vi "NormalToHex.vi"(11 "Input":string="1234") -> (3 "Output":string)   [LabVIEW 2013, in "main.lvlib"]
uses:
  main.lvlib
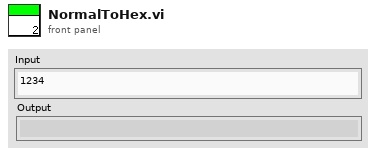
[diagram p1: front panel]
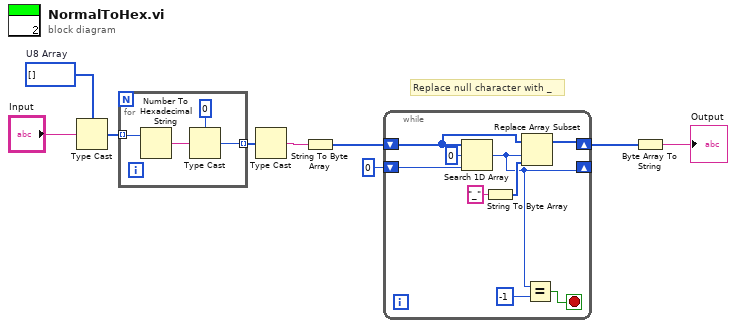
[diagram p0: block diagram]
diagram:
  w9 = u8[] []  # U8 Array
  # "Replace null character with _"
  n1 = Type Cast(type=w9, x="Input") -> (*(type *) &x=w8:u8[])
  n2 = for {
    tunnel: w8 -> [w13] mode=indexing
    tunnel: [w10] -> w7 mode=indexing
    n3 = Number To Hexadecimal String(2:w13) -> (0:w12:string)  [unwired: 1 in]
    n4 = Type Cast(type=u16 0, x=w12) -> (*(type *) &x=w10:u16)
  }
  n5 = Type Cast(x=w7) -> (*(type *) &x=w2:string)  [unwired: 1 in]
  n6 = String To Byte Array(string=w2) -> (unsigned byte array=w5:u8[])
  n7 = while {
    shift-right: [w18] -> w4
    shift-left: w5 -> [w21]
    shift-right: [w15] -> _
    shift-left: 0 ("index of element") -> [w17]
    stop <- w16 stop-if-true
    n8 = Search 1D Array(1D array=w21, element=u8 0, start index (0)=w17) -> (index of element=w15:i32)
    n9 = String To Byte Array(string="_") -> (unsigned byte array=w19:u8[])
    n10 = Replace Array Subset(array=w21, new element=w19, index=w15) -> (w18:u8[])
    n11 = Equal?(x=w15, y=-1) -> (x = y?=w16:bool)
  }
  n12 = Byte Array To String(unsigned byte array=w4) -> (string=→"Output":string)
